vi "PCSMain.constructor.vi"(0 "name":string, 2 "data in":string, 5 "error in":errorcluster) -> (14 "i ref out":refnum<vi>, 16 "data out":string, 19 "error out":errorcluster)   [LabVIEW 2014, in "PCSMain.lvlib"]
doc: "This class is forseen to select PHELIX devices to work with. Therefore it reads the data base. It also opens a connection to other PCS nodes.\n\nThis class is part of the PHELIX user layer.\n\nauthor: Stefan Götte, GSI\n\nLicense Agreement for this software:\n\nCopyright (C)\nGesellschaft für Schwerionenforschung, GSI\nPlanckstr. 1\n64291 Darmstadt\nGermany\n\nContact: D.Beck@gsi.de \n\nThis program is free software; you can redistribute it and/or modify it under the terms of the \nGNU General Public License as published by the Free Software Foundation; either version 2 of \nthe license, or (at your option) any later version.\n\nThis program is distributed in the hope that it will be useful, but WITHOUT ANY WARRANTY; \nwithout even the implied warranty of MERCHANTABILITY or FITNESS FOR A PARTICULAR PURPOSE. See the GNU General License for more details (http://www.gnu.org).\n\nGesellschaft für Schwerionenforschung, GSI\nPlanckstr. 1, 64291 Darmstadt, Germany\nFor all questions and ideas contact: M.Richter@gsi.de, H.Brand@gsi.de or D.Beck@gsi.de.\nLast update: 16-JUN-2004"
uses:
  PCSMain.lvlib
  CSCore/BaseGUI/BaseGUI.lvlib
  CSCore/CSObj/CSObj.lvlib
  CSCore/CSSystem/CSSystemLib/CSSystemLib.lvlib
  PH_Common/PH_Common.lvlib
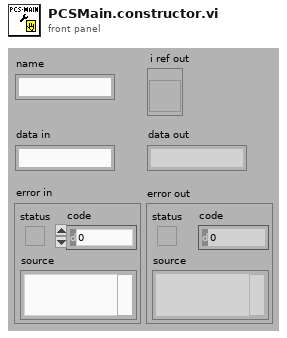
[diagram p1: front panel]
types:
  T1 = enum16{"SetAttribute", "GetAttribute", "CreateAttribute", "DestroyAttribute", "DestroyAllAtributes"}
  T2 = typedef "PCSMain.lvlib/PCSMain.i attribute.ctl" = cluster{"System Objects":cluster{"Spectrometer Objects":string[], "Camera Objects":string[], "Image Operator Objects":string[], "Gate- and Delaygenerators":string[], "Current Meas Objects":string[], "Calorimeter Objects":string[], "Powermeter Objects":string[], "SSAC Objects":string[], "Vacuum Control Objects":string[], "Countdown Counter Objects":string[], "Beckhoff Watchdog Objects":string[], "SHS Analyzer Objects":string[]}, "Local Objects":cluster{"Spectrometer Objects":string[], "Camera Objects":string[], "Image Operator Objects":string[], "Gate- and Delaygenerators":string[], "Current Meas Objects":string[], "Calorimeter Objects":string[], "Powermeter Objects":string[], "SSAC Objects":string[], "Vacuum Control Objects":string[], "Countdown Counter Objects":string[], "Beckhoff Watchdog Objects":string[], "SHS Analyzer Objects":string[]}, "Systems on same node":string[], "Data Viewer visible?":bool, "Running Objects":cluster{"Operators":bool, "SHS Analyzers":bool}, "Cam Instance System ID":string, "Black Box Objects":string[], "Switch Objects":string[], "Motion GUI Objects":string[], "Osci Objects":string[]}
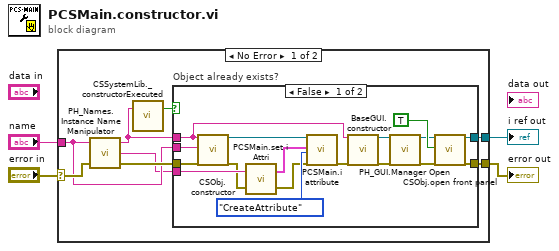
[diagram p0: block diagram]
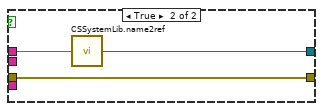
[diagram p2: hidden frame]
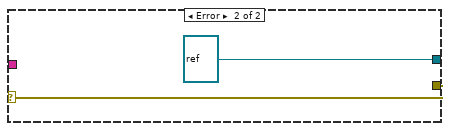
[diagram p3: hidden frame]
diagram:
  n1 = case shown="No Error" "error in" {
    selector: "error in" -> [w9 w34]
    tunnel: "name" -> [w7 _]
    tunnel: [w12 refnum<vi> refnum ("i ref out")] -> w3
    tunnel: [w11 w34] -> w2
    frame No Error {
      n2 = call "PH_Names.Instance Name Manipulator.vi"("error in (no error)"=w9, "name in"=w7) -> ("error out"=w8:errorcluster, "systemID"=w5:string, "name out"=w6:string)  [unwired: 1 in]
      n3 = call "CSSystemLib._constructorExecuted.vi"("name"=w6) -> ("constructor executed?"=w10:bool)  [unwired: 18 in]
      n4 = case "Object already exists?" shown="False" w10 {
        tunnel: w6 -> [w27 w31]
        tunnel: w8 -> [w26 w32]
        tunnel: w7 -> [w25 _]
        tunnel: [w22 w30] -> w12
        tunnel: [w23 w32] -> w11
        tunnel: w5 -> [w20 _]
        frame False {
          n5 = call "CSObj.constructor.vi"("name"=w27, "data in"=w25, "error in (no error)"=w26) -> ("i ref out"=w28:refnum<vi>, "error out"=w18:errorcluster)  [unwired: 14 in, 1 out]
          n6 = call "PCSMain.set i Attri.vi"("error in (no error)"=w18, "systemID"=w20) -> ("error out"=w17:errorcluster, "i attribute"=w19:T2)
          n7 = call "PCSMain.i attribute.vi"("VI Refnum"=w28, "CLASS.i attribute"=w19, "Action"=T1."CreateAttribute", "error in (no error)"=w17) -> ("error out"=w21:errorcluster)  [unwired: 13 in, 2 out]
          n8 = call "BaseGUI.constructor.vi"("name"=w27, "error in (no error)"=w21) -> ("i ref out"=w14:refnum<vi>, "error out"=w13:errorcluster)  [unwired: 15 in, 1 out]
          n9 = call "PH_GUI.Manager Open.vi"("i ref in"=w14, "error in"=w13) -> ("i ref out"=w16:refnum<vi>, "error out"=w15:errorcluster)  [unwired: 16 in]
          n10 = call "CSObj.open front panel.vi"("i ref in"=w16, "frontPanelOpen"=TRUE ("front panel open"), "error in (no error)"=w15) -> ("i ref out"=w22:refnum<vi>, "error out"=w23:errorcluster)  [unwired: 15 in]
        }
        frame True {
          n11 = call "CSSystemLib.name2ref.vi"("name"=w31) -> ("obj refnum"=w30:refnum<vi>)
        }
      }
    }
    frame Error {
    }
  }
  "i ref out" <- w3
  "error out" <- w2
